vi "Simulate_Gaussian.vi"(9 "Noise":dbl=10.0, 10 "Simulation":dbl[](array[slide])=[97.19626168224299, 146.41744548286604, 94.70404984423675, 22.429906542056074, 38.006230529595015, 104.04984423676012] caption="Amplitude\n\n\nX-Position\n\n\nY-Position\n\n\nWidth A\n\n\nWidth B\n\n\nAngle" scale=0.0..200.0, 11 "Sim Dim.":cluster{"Width":dbl, "Height":dbl}) -> (3 "OD(2D)":dbl[][](array[numeric]))   [LabVIEW 2015]
uses:
  <vilib>/Analysis/NI_AALBase.lvlib
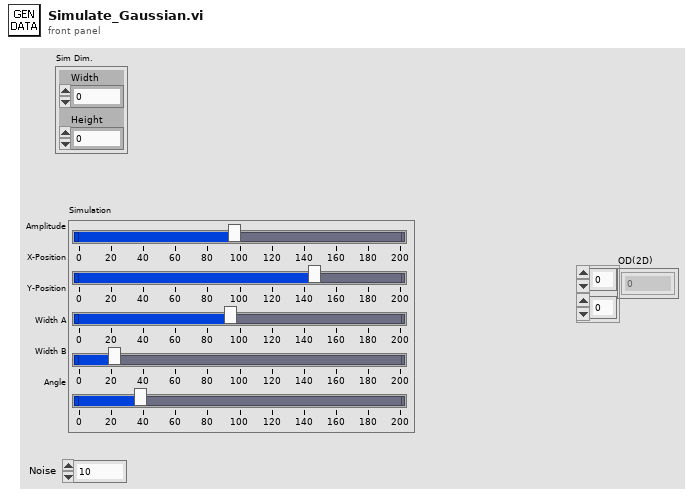
[diagram p1: front panel]
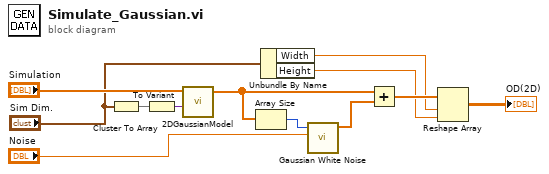
[diagram p0: block diagram]
diagram:
  n1 = Cluster To Array(cluster="Sim Dim.") -> (array=w1:dbl[])
  n2 = To Variant(anything=w1) -> (Variant=w8:variant)
  n3 = call "2DGaussianModel.vi"("data"=w8, "a"="Simulation") -> ("f(X,a)"=w6:dbl[])  [unwired: 2 in, 2 out]
  n4 = Array Size(array=w6) -> (size(s)=w10:i32)
  n5 = Unbundle By Name("Sim Dim.") -> ("Width"=w5:dbl, "Height"=w4:dbl)
  n6 = call <vilib>:"Gaussian White Noise.vi"("standard deviation"="Noise", "samples"=w10) -> ("Gaussian noise pattern"=w12:dbl[])  [unwired: 8 in, 1 out]
  n7 = Add(x=w6, y=w12) -> (x+y=w9:dbl[])
  n8 = Reshape Array(w9, w5, w4) -> (→"OD(2D)":dbl[][])
